vi "MBinteractive_while.vi"(0 "object in":refnum<class "MBinteractive.lvclass">, 5 "error in (no error)":errorcluster) -> (14 "object out":refnum<class "MBinteractive.lvclass">, 19 "error out":errorcluster)   [LabVIEW 2016, in "MBinteractive.lvclass"]
uses:
  MBinteractive.lvclass
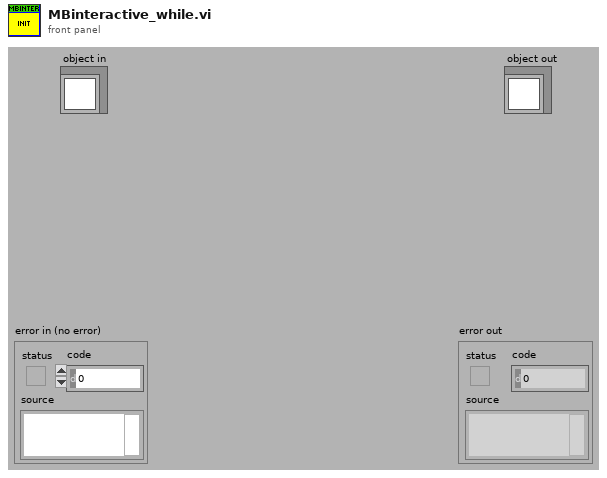
[diagram p1: front panel]
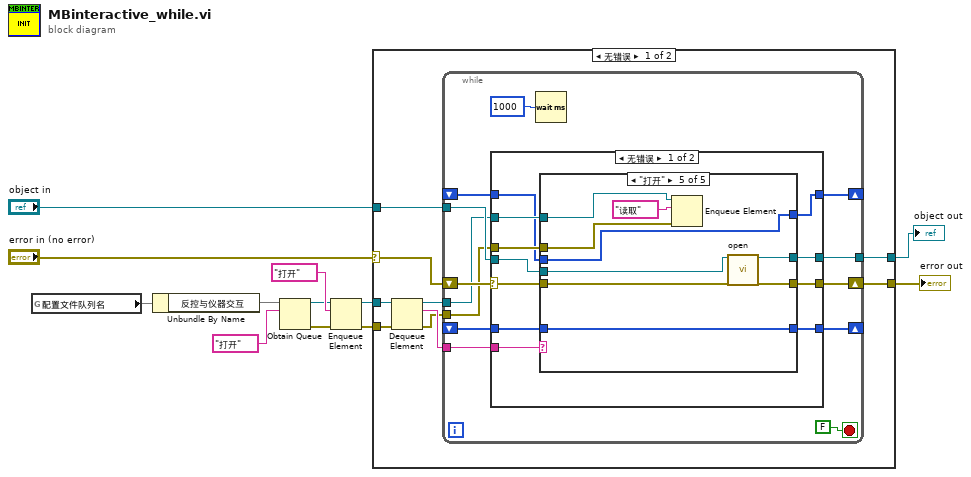
[diagram p0: block diagram]
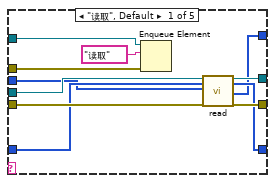
[diagram p2: hidden frame]
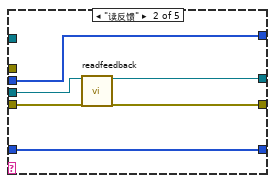
[diagram p3: hidden frame]
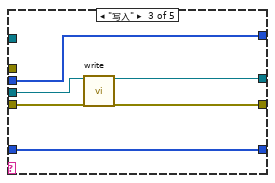
[diagram p4: hidden frame]
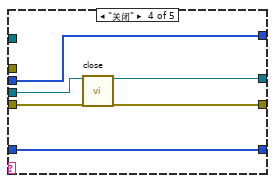
[diagram p5: hidden frame]
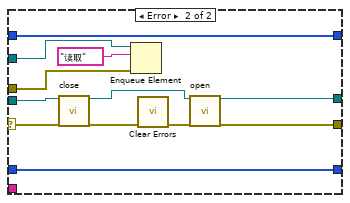
[diagram p6: hidden frame]
diagram:
  n1 = global read "断电保存全局.vi" "配置文件队列名"() -> (w3)
  n2 = Unbundle By Name(w3) -> ("反控与仪器交互"=w4)
  n3 = Obtain Queue(name (unnamed)=w4, element data type="打开" ("读取写入选择")) -> (queue out=w6:refnum<queue>, error out=w7:errorcluster)  [unwired: 3 in, 1 out]
  n4 = Enqueue Element(queue=w6, element="打开" ("读取写入选择"), error in (no error)=w7) -> (queue out=w2:refnum<queue>, error out=w1:errorcluster)  [unwired: 1 in, 1 out]
  n5 = case shown="无错误" "error in (no error)" {
    selector: "error in (no error)" -> [w18 w96]
    tunnel: [w15 w97] -> w12
    tunnel: "object in" -> [w16 w97]
    tunnel: [w17 w96] -> w9
    tunnel: w2 -> [w21 _]
    tunnel: w1 -> [w20 _]
    frame No Error {
      n6 = Dequeue Element(queue=w21, error in (no error)=w20) -> (queue out=w14:refnum<queue>, element=w19:string, error out=w13:errorcluster)  [unwired: 1 in, 1 out]
      n7 = while {
        tunnel: w19 -> [w32]
        shift-right: [w29] -> w17
        shift-left: w18 -> [w28]
        tunnel: w16 -> [w31]
        tunnel: [w30] -> w15
        tunnel: w14 -> [w27]
        tunnel: w13 -> [w26]
        shift-right: [w25] -> _
        shift-left: _ -> [w24]
        shift-right: [w23] -> _
        shift-left: _ -> [w22]
        stop <- FALSE stop-if-true
        n8 = case shown="无错误" w28 {
          selector: w28 -> [w41 w94]
          tunnel: w32 -> [w45 _]
          tunnel: w31 -> [w44 w95]
          tunnel: [w43 w89] -> w30
          tunnel: [w42 w91] -> w29
          tunnel: w27 -> [w40 w87]
          tunnel: w26 -> [w39 w86]
          tunnel: [w38 w85] -> w25
          tunnel: w24 -> [w37 w85]
          tunnel: [w36 w84] -> w23
          tunnel: w22 -> [w35 w84]
          frame No Error {
            n9 = case shown="\"打开\"" w45 {
              tunnel: w44 -> [w56 w61 w68 w74 w83]
              tunnel: [w55 w59 w65 w71 w81] -> w43
              tunnel: w41 -> [w54 w62 w67 w73 w82]
              tunnel: [w53 w60 w66 w72 w80] -> w42
              tunnel: w40 -> [w51 _ _ _ w79]
              tunnel: w39 -> [w50 _ _ _ w78]
              tunnel: [w49 w58 w64 w70 w76] -> w38
              tunnel: w37 -> [w48 w58 w64 w70 w76]
              tunnel: [w47 w57 w63 w69 w75] -> w36
              tunnel: w35 -> [w46 w57 w63 w69 w75]
              frame "读取", Default {
                n10 = Enqueue Element(queue=w51, element="读取" ("读取写入选择"), error in (no error)=w50) -> ()  [unwired: 1 in, 3 out]
                n11 = call-dynamic "read.vi"("object in"=w56, "上次仪器状态"=w48, "上次各参数测量间隔"=w46, "error in (no error)"=w54) -> ("object out"=w55:refnum<class "MBinteractive.lvclass">, "仪器状态"=w49:u16[], "各参数测量间隔"=w47:u16[], "error out"=w53:errorcluster)  [unwired: 12 in]
              }
              frame "读反馈" {
                n12 = call-dynamic "readfeedback.vi"("object in"=w61, "error in (no error)"=w62) -> ("object out"=w59:refnum<class "MBinteractive.lvclass">, "error out"=w60:errorcluster)  [unwired: 15 in, 1 out]
              }
              frame "写入" {
                n13 = call-dynamic "write.vi"("object in"=w68, "error in (no error)"=w67) -> ("object out"=w65:refnum<class "MBinteractive.lvclass">, "error out"=w66:errorcluster)  [unwired: 16 in]
              }
              frame "关闭" {
                n14 = call-dynamic "close.vi"("object in"=w74, "error in (no error)"=w73) -> ("object out"=w71:refnum<class "MBinteractive.lvclass">, "error out"=w72:errorcluster)  [unwired: 16 in]
              }
              frame "打开" {
                n15 = Enqueue Element(queue=w79, element="读取" ("读取写入选择"), error in (no error)=w78) -> ()  [unwired: 1 in, 3 out]
                n16 = call-dynamic "open.vi"("object in"=w83, "error in (no error)"=w82) -> ("object out"=w81:refnum<class "MBinteractive.lvclass">, "error out"=w80:errorcluster)  [unwired: 16 in]
              }
            }
          }
          frame Error {
            n17 = call-dynamic "close.vi"("object in"=w95, "error in (no error)"=w94) -> ("object out"=w90:refnum<class "MBinteractive.lvclass">, "error out"=w93:errorcluster)  [unwired: 16 in]
            n18 = Enqueue Element(queue=w87, element="读取" ("读取写入选择"), error in (no error)=w86) -> ()  [unwired: 1 in, 3 out]
            n19 = call <vilib>:"Clear Errors.vi"("error in (no error)"=w93) -> ("error out"=w92:errorcluster)  [unwired: 5 in, 1 out]
            n20 = call-dynamic "open.vi"("object in"=w90, "error in (no error)"=w92) -> ("object out"=w89:refnum<class "MBinteractive.lvclass">, "error out"=w91:errorcluster)  [unwired: 16 in]
          }
        }
        n21 = Wait (ms)(milliseconds to wait=u32 1000 ("等待时间（毫秒）")) -> ()  [unwired: 1 out]
      }
    }
    frame Error {
    }
  }
  "object out" <- w12
  "error out" <- w9
